vi "Sweep Field and Get Data.vi"(4 "error in":errorcluster, 5 "Spectral Data In":T1={"PDT Amp [v]"=0.0, "RIS Amp [v]"=0.0, "B-Field"=[], "All In-Phase Scan Spectra"=[], "Model Select"=enum."OneCompRISTwoPDT", "Fit Each Scan"=FALSE, "PDT Center [g]"=0.0, "In-Phase Average Spectra"=[], "In-Phase Median Spectra"=[], "Out-Phase Median Spectra"=[], "Out-Phase Average Spectra"=[], "Fit Spectra"=[], "Fit No-Baseline Spectra"=[], "All Out-Phase Scan Spectra"=[], "Baseline Offset Correction"=FALSE, "In-Phase Offset [v]"=0.0, "Out-Phase Offset [v]"=0.0, "Ch2 Input\n(Balance)"=[], "Ch3 Input\n(Phase)"=[], "Ch4 Input\n(AFC)"=[], "Fit Pars"=[], "Fit Pars Errors"=[], "Fit Pars Labels"=[], "Raw Scan DAQ Data"=[], "Bad Scans Indicies"=[], "Good In-Phase Scan Spectra"=[], "Good Out-Phase Scan Spectra"=[], "Bad In-Phase Scan Spectra"=[], "Bad Out-Phase Scan Spectra"=[], "Number of bad scans"=0, "Fit History"=[], "PDT Amp. History/Set [v]"=[], "RIS Amp. History/Set [v]"=[], "RIS Amp. History/Scan [v]"=[], "All Shifted B-Fields"=[], "Good Shifted B-Fields"=[], "Ch5 Input\n(SpO2)"=[], "Ch6 Input\n(BPM)"=[], "Global SNR"=0.0, "Fit Error History"=[], "SNR History"=[]} {"Global SNR" min=0.0; "PDT Center [g]" min=0.0; "RIS Amp [v]" min=0.0; "PDT Amp [v]" min=0.0}, 6 "Hardware Parameters":T3={"Scan Calibration [G/V]"=0.0, "Modulation Calibration [G/V]"=0.0, "Modulation Phase [deg]"=0.0, "Modulation Frequency [Hz]"=0.0, "Attenuation [dB]"=0, "Input Channel Count"=0, "Time constant"=7, "Sensitivity"=17, "Frequency Output Voltage [V]"=0.0, "Phase Output Voltage [V]"=0.0, "Lock-in Offset Compensation"=FALSE, "RF [GHz]"=0.0, "Q Start"=0.0, "Q End"=0.0, "Balance"=0.0, "Phase Error"=0.0, "AFC Error"=0.0, "AFC"=FALSE, "Magnet Rotation"=FALSE, "Balance Scaling Factor"=1.0, "Phase Error Scaling Factor"=1.0, "AFC Error Scaling Factor"=1.0, "Frequency Counter ID"="", "Sweep Waveform"=enum."Sawtooth", "Q-Factor Scale"=0.0, " Q-Data Scale"=0.0, " Q-Data Offset"=0.0, "Magnet Rotation Slope"=0.0, "Magnet Rotation Offset"=0.0, "Phase Sweep Resolution"=0.0, "Hardware Version Number"="", "Spectrometer ID Number"=0, "Spectrometer Name"="", "Lock in Saturation"=0.0, "Balance Threshold"=0.0, "Phase Error Threshold"=0.0, "AFC Error Threshold"=0.0, "Linear Actuator Length"=0.0, "Lock-in OK?"=FALSE, "Ignore Lock-in Comm. Failure"=FALSE, "Gradient Addresses"=[], "Gradient Calibrations [G/A*mm]"=[], "Gradient Power Supplies"=[], "Lock-in Address"="", "Magnet Type"=enum."RRI", "Camera Names"=[], "Sweep Limit [Gauss]"=0.0, "Modulation Limit [Gauss]"=0.0, "Balance Threshold Exceeded?"=FALSE, "Phase Threshold Exceeded?"=FALSE, "AFC Threshold Exceeded?"=FALSE, "Consecutive Re-tune attempts"=0, "Reverse Sweep Slope [sec]"=0.0, "Reverse Sweep Offset [G]"=0.0, "AFC Field Correction [V/MHz]"=0.0, "Active Gradients (X Y Z)"=[], "SpO2 Calibration [SpO2/V]"=1.0, "Heart Rate Calibration [BPM/V]"=1.0, "Thermocouple Channel"=""} {"Sensitivity" items=["10 us", "20 us", "40 us", "80 us", "160 us", "320 us", "640 us", "5 ms", "10 ms", "20 ms", "50 ms", "100 ms", "200 ms", "500 ms", "1 s", "2 s", "5 s", "10 s", "20 s", "50 s", "100 s", "200 s", "500 s", "1 ks", "2 ks", "5 ks", "10 ks", "20 ks", "50 ks", "100 ks"]; "Time constant" items=["10 us", "20 us", "40 us", "80 us", "160 us", "320 us", "640 us", "5 ms", "10 ms", "20 ms", "50 ms", "100 ms", "200 ms", "500 ms", "1 s", "2 s", "5 s", "10 s", "20 s", "50 s", "100 s", "200 s", "500 s", "1 ks", "2 ks", "5 ks", "10 ks", "20 ks", "50 ks", "100 ks"]}, 7 "Acquisition Parameters":T4={"Magnet Angle [deg]"=0.0, "Magnet Angles [deg]"=[], "DeltaVpp [v]"=0.0, "SEM [v]"=0.0, "DeltaVpp Thresh [v]"=0.0, "SEM Thresh [v]"=0.0, "Adaptive Processing"=FALSE, "Acquire Q"=FALSE, "Acquire Photos"=FALSE, "Adaptive Tuning"=FALSE, "Automated Matching"=FALSE, "X-Gradient [G/mm]"=0.0, "Y-Gradient [G/mm]"=0.0, "Z-Gradient [G/mm]"=0.0, "Central Field [G]"=0.0, "Scan Width [G]"=0.0, "Mod. Amp. [G]"=0.0, "Scan Time [s]"=0.0, "Pre-Scan Delay [ms]"=0, "Measurement Timeout [s]"=0.0, "Electromagnet Main Field [G]"=0.0, "Locked Central Field [G]"=0.0, "Scans Excluded"=0, "Scans Completed"=0, "No. Scans/Set"=0, "No. Scans for SNR"=0, "Field Locked Frequency [GHz]"=0.0, "Auto Set-based Field Center"=FALSE, "Prompt for oxy acquisition updates"=FALSE, "Oxy QA Scan?"=FALSE, "Exclude Bad Data"=FALSE, "Optimizing RF Power"=FALSE, "Gradients on/off"=FALSE, "Running Script"=TRUE, "Opto-Coupler Current [A]"=0.0, "Continuous Sweeping"=FALSE, "Sweep Rise Time [sec]"=0, "Reverse Sweep Central Field [G]"=0.0, "Forward Sweep Central Field [G]"=0.0, "Sweep Calibrated"=FALSE, "Modulation Calibrated"=FALSE, "First CheckCal Scan?"=FALSE, "AFC Field Correction"=FALSE, "OxyQAInit Scan Width [G]"=0.0, "OxyQAInit Mod. Amp. [G]"=0.0, "Scans Completed/Session"=0, "Acquire SpO2"=FALSE, "Acquire Temperature"=FALSE, "Over Mod"=FALSE} {"OxyQAInit Mod. Amp. [G]" min=0.0; "OxyQAInit Scan Width [G]" min=0.0; "Mod. Amp. [G]" min=0.0; "Scan Width [G]" min=0.0; "Central Field [G]" min=0.0; "Measurement Timeout [s]" min=0.0; "Scan Time [s]" min=0.0; "Z-Gradient [G/mm]" min=0.0; "SEM [v]" min=0.0; "DeltaVpp [v]" min=0.0}) -> (0 "error out":errorcluster, 2 "Raw DAQ Data Out":dbl[][](array[numeric]), 3 "Spectral Data Out":T1={"PDT Amp [v]"=0.0, "RIS Amp [v]"=0.0, "B-Field"=[], "All In-Phase Scan Spectra"=[], "Model Select"=enum."OneCompRISTwoPDT", "Fit Each Scan"=FALSE, "PDT Center [g]"=0.0, "In-Phase Average Spectra"=[], "In-Phase Median Spectra"=[], "Out-Phase Median Spectra"=[], "Out-Phase Average Spectra"=[], "Fit Spectra"=[], "Fit No-Baseline Spectra"=[], "All Out-Phase Scan Spectra"=[], "Baseline Offset Correction"=FALSE, "In-Phase Offset [v]"=0.0, "Out-Phase Offset [v]"=0.0, "Ch2 Input\n(Balance)"=[], "Ch3 Input\n(Phase)"=[], "Ch4 Input\n(AFC)"=[], "Fit Pars"=[], "Fit Pars Errors"=[], "Fit Pars Labels"=[], "Raw Scan DAQ Data"=[], "Bad Scans Indicies"=[], "Good In-Phase Scan Spectra"=[], "Good Out-Phase Scan Spectra"=[], "Bad In-Phase Scan Spectra"=[], "Bad Out-Phase Scan Spectra"=[], "Number of bad scans"=0, "Fit History"=[], "PDT Amp. History/Set [v]"=[], "RIS Amp. History/Set [v]"=[], "RIS Amp. History/Scan [v]"=[], "All Shifted B-Fields"=[], "Good Shifted B-Fields"=[], "Ch5 Input\n(SpO2)"=[], "Ch6 Input\n(BPM)"=[], "Global SNR"=0.0, "Fit Error History"=[], "SNR History"=[]} {"Global SNR" min=0.0; "PDT Center [g]" min=0.0; "RIS Amp [v]" min=0.0; "PDT Amp [v]" min=0.0})   [LabVIEW 2016]
uses:
  Types/Acquisition Parameters.ctl
  Types/Hardware Parameters.ctl
  Types/Spectral Data.ctl
  Types/Fitting Model Selection.ctl
  Das16.llb/FromEng(single).VI
  Types/Global Variables.vi
  Das16.llb/ToEng(array).vi
panel:
  out "B-Field Out":dbl[](array[numeric])
  # "Bridge I/O"
  # "Magnet Rotation"
  # "Field Calibration"
  # "Lock In Amplifier"
  # "Spectrometer Information"
  # "DAQ Settings"
  # "Gradient Coils and Field"
  # "X"
  # "Y"
  # "Z"
  # "Q-Measurements"
  # "Gradients"
  # "Field"
  # "Scans and Sets"
  # "Timing"
  # "Adaptive Dosimetric \nData Processing"
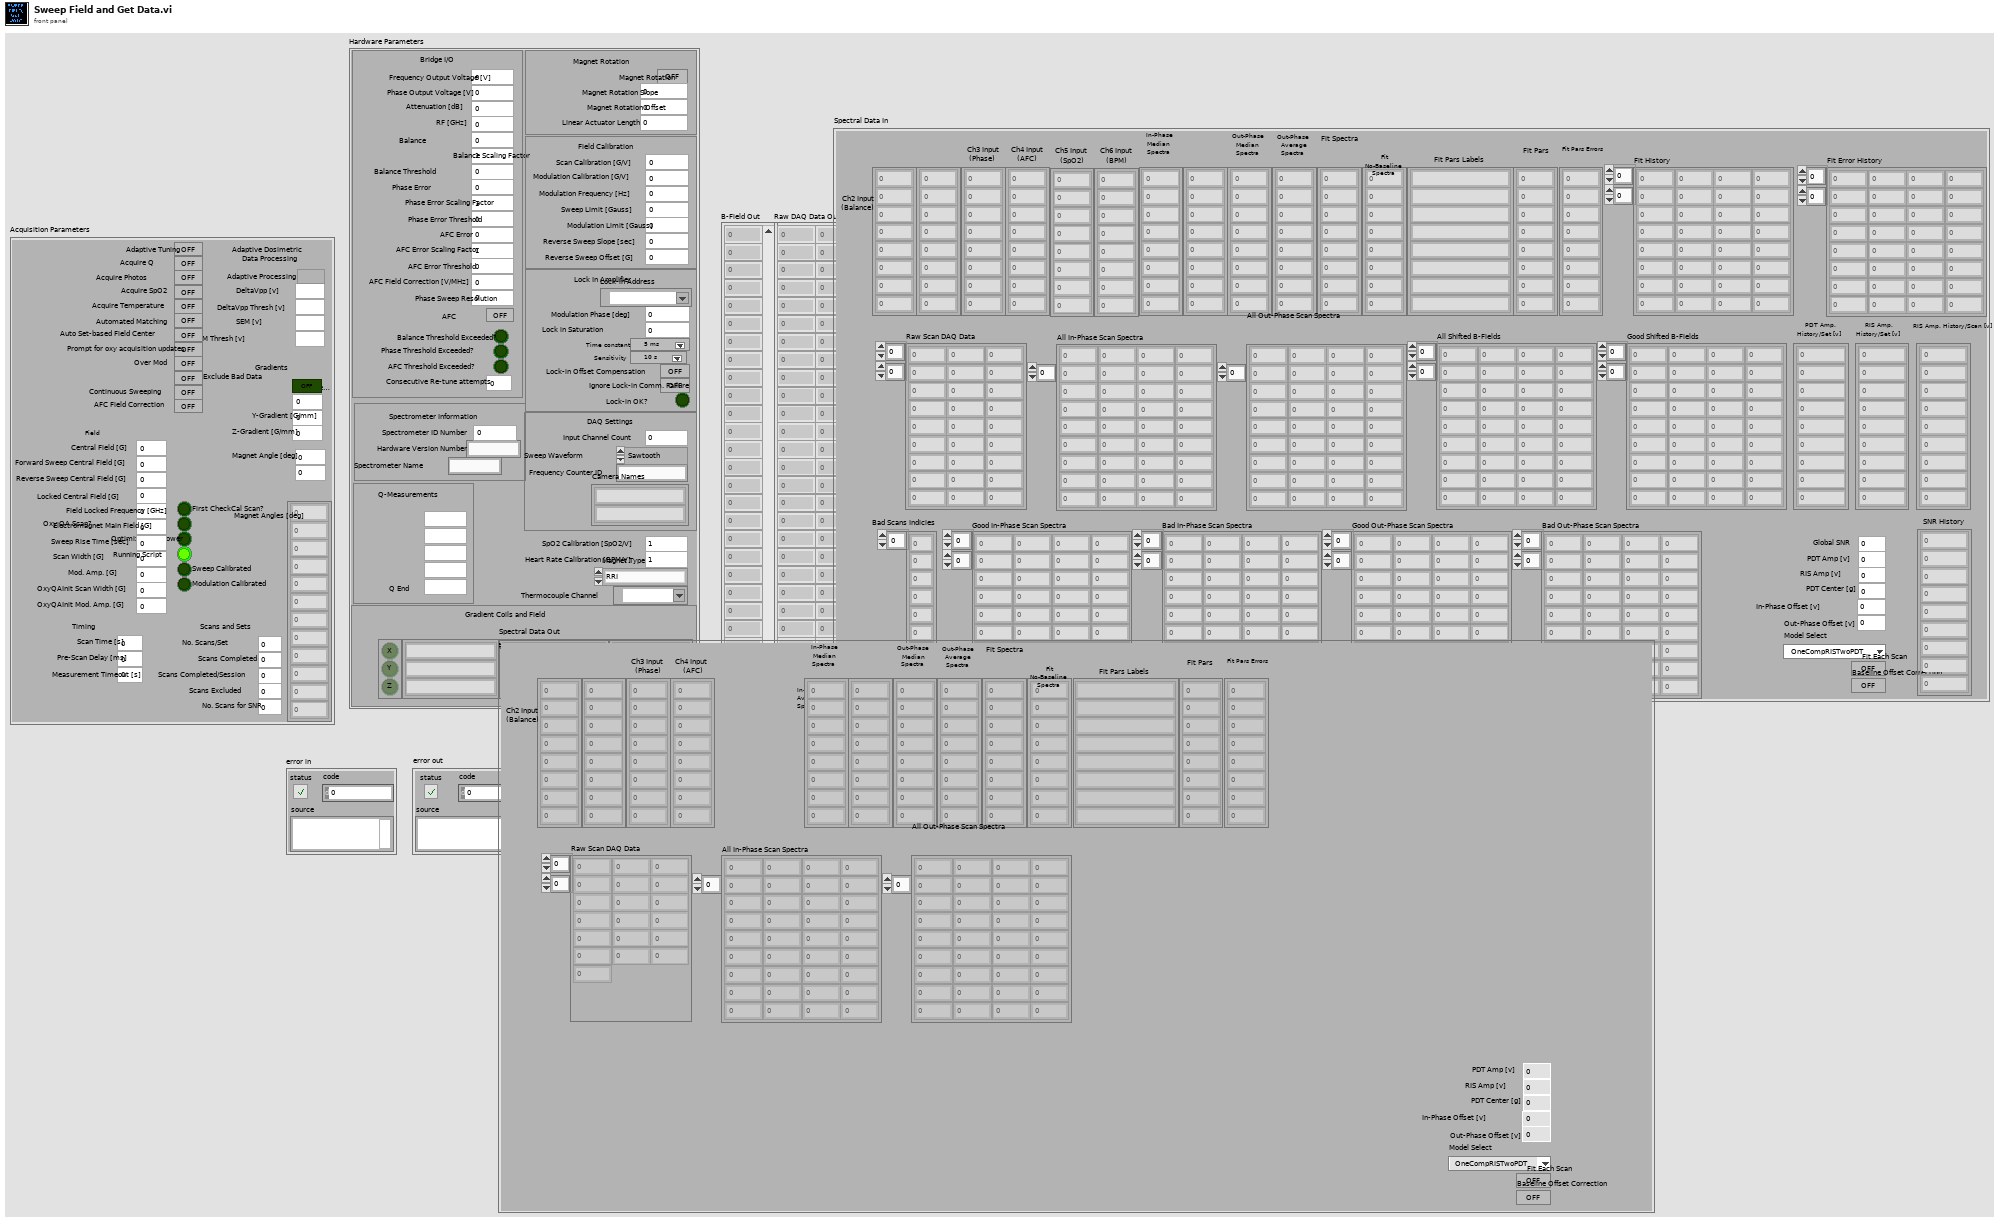
[diagram p1: front panel]
types:
  T1 = typedef "Spectral Data.ctl" = cluster{"PDT Amp [v]":dbl, "RIS Amp [v]":dbl, "B-Field":dbl[], "All In-Phase Scan Spectra":dbl[][], "Model Select":T2, "Fit Each Scan":bool, "PDT Center [g]":dbl, "In-Phase Average Spectra":dbl[], "In-Phase Median Spectra":dbl[], "Out-Phase Median Spectra":dbl[], "Out-Phase Average Spectra":dbl[], "Fit Spectra":dbl[], "Fit No-Baseline Spectra":dbl[], "All Out-Phase Scan Spectra":dbl[][], "Baseline Offset Correction":bool, "In-Phase Offset [v]":dbl, "Out-Phase Offset [v]":dbl, "Ch2 Input\n(Balance)":dbl[], "Ch3 Input\n(Phase)":dbl[], "Ch4 Input\n(AFC)":dbl[], "Fit Pars":dbl[], "Fit Pars Errors":dbl[], "Fit Pars Labels":string[], "Raw Scan DAQ Data":dbl[][], "Bad Scans Indicies":i32[], "Good In-Phase Scan Spectra":dbl[][], "Good Out-Phase Scan Spectra":dbl[][], "Bad In-Phase Scan Spectra":dbl[][], "Bad Out-Phase Scan Spectra":dbl[][], "Number of bad scans":i32, "Fit History":dbl[][], "PDT Amp. History/Set [v]":dbl[], "RIS Amp. History/Set [v]":dbl[], "RIS Amp. History/Scan [v]":dbl[], "All Shifted B-Fields":dbl[][], "Good Shifted B-Fields":dbl[][], "Ch5 Input\n(SpO2)":dbl[], "Ch6 Input\n(BPM)":dbl[], "Global SNR":dbl, "Fit Error History":dbl[][], "SNR History":dbl[]}
  T2 = typedef "Fitting Model Selection.ctl" = enum16{"OneCompRIS", "OneCompRISTwoPDT", "OneCompRISRev", "OneCompRISTwoPDTRev", "LiPc", "TwoLiPc", "ThreeLiPc", "FourLiPc", "PDTCalibration", "CE_Ink", "Printex", "MelaninTwoPDT"}
  T3 = typedef "Hardware Parameters.ctl" = cluster{"Scan Calibration [G/V]":dbl, "Modulation Calibration [G/V]":dbl, "Modulation Phase [deg]":dbl, "Modulation Frequency [Hz]":dbl, "Attenuation [dB]":u16, "Input Channel Count":i32, "Time constant":u16, "Sensitivity":u16, "Frequency Output Voltage [V]":dbl, "Phase Output Voltage [V]":dbl, "Lock-in Offset Compensation":bool, "RF [GHz]":dbl, "Q Start":dbl, "Q End":dbl, "Balance":dbl, "Phase Error":dbl, "AFC Error":dbl, "AFC":bool, "Magnet Rotation":bool, "Balance Scaling Factor":dbl, "Phase Error Scaling Factor":dbl, "AFC Error Scaling Factor":dbl, "Frequency Counter ID":string, "Sweep Waveform":enum16{"Sine Wave", "Square Wave", "Sawtooth", "Triangle Wave"}, "Q-Factor Scale":dbl, " Q-Data Scale":dbl, " Q-Data Offset":dbl, "Magnet Rotation Slope":dbl, "Magnet Rotation Offset":dbl, "Phase Sweep Resolution":dbl, "Hardware Version Number":string, "Spectrometer ID Number":i32, "Spectrometer Name":string, "Lock in Saturation":dbl, "Balance Threshold":dbl, "Phase Error Threshold":dbl, "AFC Error Threshold":dbl, "Linear Actuator Length":dbl, "Lock-in OK?":bool, "Ignore Lock-in Comm. Failure":bool, "Gradient Addresses":string[], "Gradient Calibrations [G/A*mm]":dbl[], "Gradient Power Supplies":string[], "Lock-in Address":refnum<visa-resource-name>, "Magnet Type":enum16{"RRI", "BARDA", "Whole Body Permanent", "RRI Electromagnet"}, "Camera Names":string[], "Sweep Limit [Gauss]":dbl, "Modulation Limit [Gauss]":dbl, "Balance Threshold Exceeded?":bool, "Phase Threshold Exceeded?":bool, "AFC Threshold Exceeded?":bool, "Consecutive Re-tune attempts":i32, "Reverse Sweep Slope [sec]":dbl, "Reverse Sweep Offset [G]":dbl, "AFC Field Correction [V/MHz]":dbl, "Active Gradients (X Y Z)":bool[], "SpO2 Calibration [SpO2/V]":dbl, "Heart Rate Calibration [BPM/V]":dbl, "Thermocouple Channel":tag}
  T4 = typedef "Acquisition Parameters.ctl" = cluster{"Magnet Angle [deg]":dbl, "Magnet Angles [deg]":dbl[], "DeltaVpp [v]":dbl, "SEM [v]":dbl, "DeltaVpp Thresh [v]":dbl, "SEM Thresh [v]":dbl, "Adaptive Processing":bool, "Acquire Q":bool, "Acquire Photos":bool, "Adaptive Tuning":bool, "Automated Matching":bool, "X-Gradient [G/mm]":dbl, "Y-Gradient [G/mm]":dbl, "Z-Gradient [G/mm]":dbl, "Central Field [G]":dbl, "Scan Width [G]":dbl, "Mod. Amp. [G]":dbl, "Scan Time [s]":dbl, "Pre-Scan Delay [ms]":u32, "Measurement Timeout [s]":dbl, "Electromagnet Main Field [G]":dbl, "Locked Central Field [G]":dbl, "Scans Excluded":u32, "Scans Completed":u32, "No. Scans/Set":u32, "No. Scans for SNR":u32, "Field Locked Frequency [GHz]":dbl, "Auto Set-based Field Center":bool, "Prompt for oxy acquisition updates":bool, "Oxy QA Scan?":bool, "Exclude Bad Data":bool, "Optimizing RF Power":bool, "Gradients on/off":bool, "Running Script":bool, "Opto-Coupler Current [A]":dbl, "Continuous Sweeping":bool, "Sweep Rise Time [sec]":u32, "Reverse Sweep Central Field [G]":dbl, "Forward Sweep Central Field [G]":dbl, "Sweep Calibrated":bool, "Modulation Calibrated":bool, "First CheckCal Scan?":bool, "AFC Field Correction":bool, "OxyQAInit Scan Width [G]":dbl, "OxyQAInit Mod. Amp. [G]":dbl, "Scans Completed/Session":u32, "Acquire SpO2":bool, "Acquire Temperature":bool, "Over Mod":bool}
  T5 = enum16{"Sine Wave", "Square Wave", "Sawtooth", "Triangle Wave"}
  T6 = cluster{"IntnlBoardNum":i32, "Data":i16[], "Size":i32, "IntnlStatus":i32, "IntnlErrCode":i32, "Alias16":u32, "Reserved":i32}
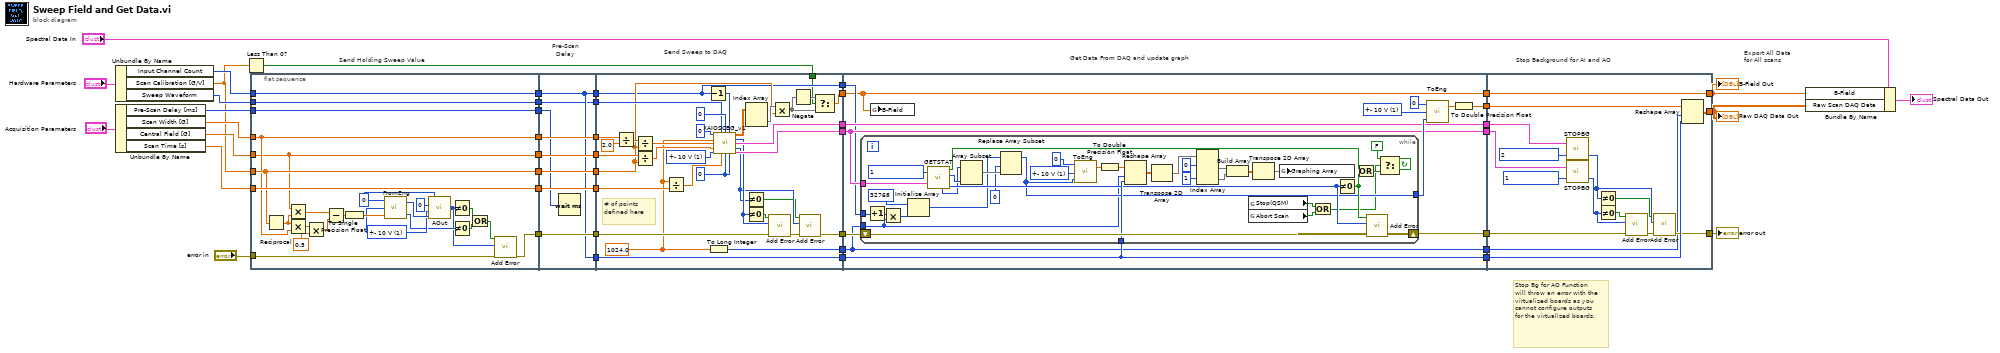
[diagram p0: block diagram]
diagram:
  # "Stop Background for AI and AO"
  # "Get Data From DAQ and update graph"
  # "Send Holding Sweep Value"
  # "Pre-Scan\n  Delay"
  # "Send Sweep to DAQ"
  # "Stop Bg for AO Function will throw an error with the virtualized boards as you cannot configure outputs for the virtualized boards."
  # "Export All Data \nfor All scans"
  n1 = Unbundle By Name("Hardware Parameters") -> ("Input Channel Count"=w16:i32, "Scan Calibration [G/V]"=w2:dbl, "Sweep Waveform"=w12:T5)
  n2 = Unbundle By Name("Acquisition Parameters") -> ("Pre-Scan Delay [ms]"=w17:u32, "Scan Width [G]"=w15:dbl, "Central Field [G]"=w14:dbl, "Scan Time [s]"=w13:dbl)
  n3 = Less Than 0?(x=w2) -> (x < 0?=w1:bool)
  n4 = flat-sequence {
    tunnel: w13 -> [w70]
    tunnel: w14 -> [w62]
    tunnel: w15 -> [w63]
    tunnel: w2 -> [w64]
    tunnel: "error in" -> [w54]
    tunnel: w16 -> [w71]
    tunnel: [w71] -> w46
    tunnel: [w52] -> w45
    tunnel: [w64] -> w44
    tunnel: [w63] -> w43
    tunnel: [w62] -> w42
    tunnel: [w70] -> w41
    tunnel: w17 -> [w53]
    tunnel: [w53] -> w40
    tunnel: w12 -> [w47]
    tunnel: [w47] -> w10
    tunnel: w46 -> [w73]
    tunnel: [w73] -> w39
    tunnel: w45 -> [w79]
    tunnel: [w79] -> w38
    tunnel: w44 -> [w78]
    tunnel: [w78] -> w37
    tunnel: w43 -> [w77]
    tunnel: [w77] -> w36
    tunnel: w42 -> [w76]
    tunnel: [w76] -> w35
    tunnel: w41 -> [w75]
    tunnel: [w75] -> w34
    tunnel: w40 -> [w74]
    tunnel: [w73] -> w33
    tunnel: [w72] -> w11
    tunnel: w10 -> [w72]
    tunnel: [w103] -> w32
    tunnel: [w102] -> w31
    tunnel: w39 -> [w86]
    tunnel: w38 -> [w97]
    tunnel: w37 -> [w87]
    tunnel: w36 -> [w101]
    tunnel: w35 -> [w100]
    tunnel: w34 -> [w99]
    tunnel: w33 -> [w98]
    tunnel: [w98] -> w30
    tunnel: [w93] -> w29
    tunnel: [w83] -> w28
    tunnel: w11 -> [w89]
    tunnel: [w86] -> w9
    tunnel: [w84] -> w8
    tunnel: w1 -> [w80]
    tunnel: w32 -> [w123]
    tunnel: w31 -> [w122]
    tunnel: [w123] -> w27
    tunnel: [w122] -> w26
    tunnel: [w117] -> w25
    tunnel: [w119] -> w24
    tunnel: w30 -> [w118]
    tunnel: [w118] -> w23
    tunnel: w29 -> [w121]
    tunnel: [w115] -> w22
    tunnel: w28 -> [w115]
    tunnel: w9 -> [w116]
    tunnel: w8 -> [w114]
    tunnel: [w114] -> w7
    tunnel: w27 -> [w179]
    tunnel: w26 -> [w178]
    tunnel: w25 -> [w173]
    tunnel: w24 -> [w175]
    tunnel: w23 -> [w172]
    tunnel: w22 -> [w165]
    tunnel: w7 -> [w164]
    tunnel: [w165] -> w5
    tunnel: [w174] -> w3
    tunnel: [w169] -> w20
    frame #0 {
      w56 = 1 items=["Not Programmable"=0, "+- 20 V"=27, "+- 10 V"=1, "+- 5 V"=2, "+- 4 V"=28, "+- 2.5 V"=3, "+- 2 V"=29, "+- 1.67 V"=4, "+- 1.25 V"=5, "+- 1 V"=6, "+- .625 V"=7, "+- .5 V"=8, "+- .25 V"=30, "+- .2 V"=31, "+- .1 V"=9, "+- .05 V"=10, "+- .01 V"=11, "+- .005 V"=12, "0 - 10 V"=13, "0 - 5 V"=14, "0 - 4 V"=36, "0 - 2.5 V"=15, "0 - 2 V"=16, "0 - 1.67 V"=17, "0 - 1.25 V"=18, "0 - 1 V"=19, "0 - .5 V"=32, "0 - .25 V"=33, "0 - .2 V"=34, "0 - .1 V"=20, "0 - .02 V"=35, "0 - .01 V"=21, "4 - 20 mA"=22, "2 - 10 mA"=23, "1 - 5 mA"=24, ".5 - 2.5 mA"=25, "0 - 20 mA"=26] ("Range")
      w58 = u32 0 ("BoardNum (0)")
      n5 = Reciprocal(x=w64) -> (1/x=w69:dbl)
      n6 = Multiply(x=w62, y=w69) -> (x*y=w65:dbl)
      n7 = Multiply(x=w69, y=w63) -> (x*y=w68:dbl)
      n8 = Multiply(x=w68, y=0.5) -> (x*y=w66:dbl)
      n9 = Subtract(x=w65, y=w66) -> (x-y=w60:dbl)
      n10 = To Single Precision Float(number=w60) -> (single precision float=w61:sgl)
      n11 = call-poly "FromEng.VI"("Eng Units"=w61, "Range"=w56, "BoardNum (0)"=w58) -> ("ErrCode"=w55:i32, "DA Data"=w57:u16)
      n12 = call "AOut.VI"("DataValue"=w57, "Range"=w56, "Channel"=0, "BoardNum"=w58) -> ("ErrCode"=w48:i32)
      n13 = Not Equal To 0?(x=w48) -> (x != 0?=w49:bool)
      n14 = Not Equal To 0?(x=w55) -> (x != 0?=w51:bool)
      n15 = Or(x=w49, y=w51) -> (x .or. y?=w50:bool)
      n16 = call "Add Error.vi"("error in (no error)"=w54, "error code (0)"=w48, "error?"=w50) -> ("error out"=w52:errorcluster)  [unwired: 8 in]
    }
    frame #1 {
      n17 = Wait (ms)(milliseconds to wait=w74) -> ()  [unwired: 1 out]
    }
    frame #2 {
      w85 = 1024.0 ("y")
      w104 = 0 ("LowAOChan")
      w112 = 1 items=["Not Programmable"=0, "+- 20 V"=27, "+- 10 V"=1, "+- 5 V"=2, "+- 4 V"=28, "+- 2.5 V"=3, "+- 2 V"=29, "+- 1.67 V"=4, "+- 1.25 V"=5, "+- 1 V"=6, "+- .625 V"=7, "+- .5 V"=8, "+- .25 V"=30, "+- .2 V"=31, "+- .1 V"=9, "+- .05 V"=10, "+- .01 V"=11, "+- .005 V"=12, "0 - 10 V"=13, "0 - 5 V"=14, "0 - 4 V"=36, "0 - 2.5 V"=15, "0 - 2 V"=16, "0 - 1.67 V"=17, "0 - 1.25 V"=18, "0 - 1 V"=19, "0 - .5 V"=32, "0 - .25 V"=33, "0 - .2 V"=34, "0 - .1 V"=20, "0 - .02 V"=35, "0 - .01 V"=21, "4 - 20 mA"=22, "2 - 10 mA"=23, "1 - 5 mA"=24, ".5 - 2.5 mA"=25, "0 - 20 mA"=26] ("Range")
      # "# of points defined here"
      n18 = Divide(x=w101, y=2.0) -> (x/y=w108:dbl)
      n19 = Divide(x=w108, y=w87) -> (x/y=w107:dbl)
      n20 = Divide(x=w100, y=w87) -> (x/y=w106:dbl)
      n21 = Divide(x=w85, y=w99) -> (x/y=w105:dbl)
      n22 = Decrement(x=w86) -> (x-1=w111:i32)
      n23 = To Long Integer(number=w85) -> (32bit integer=w84:i32)
      n24 = call "XAIOSCBG_v1.VI"("BoardNum"=u32 0, "signal type"=w89, "LowChan"=0, "HighChan"=w111, "number of points"=w85, "amplitude (1.0)"=w107, "offset (0.0)"=w106, "Range"=w112, "Rate"=w105, "HighAOChan"=w104, "LowAOChan"=w104) -> ("Output Array"=w90:dbl[][], "AIn-ErrCode"=w96:i32, "OutContext"=w103:T6, "AOut-ErrCode"=w95:i32, "InContext"=w102:T6)
      n25 = Not Equal To 0?(x=w95) -> (x != 0?=w92:bool)
      n26 = Not Equal To 0?(x=w96) -> (x != 0?=w91:bool)
      n27 = Index Array(array=w90) -> (element=w88:dbl[])  [unwired: 2 in]
      n28 = call "Add Error.vi"("error in (no error)"=w97, "error code (0)"=w96, "error?"=w91) -> ("error out"=w94:errorcluster)  [unwired: 8 in]
      n29 = Multiply(x=w88, y=w87) -> (x*y=w82:dbl[])
      n30 = Negate(x=w82) -> (-x=w81:dbl[])
      n31 = call "Add Error.vi"("error in (no error)"=w94, "error code (0)"=w95, "error?"=w92) -> ("error out"=w93:errorcluster)  [unwired: 8 in]
      n32 = Select(t=w81, s=w80, f=w82) -> (s? t:f=w83:dbl[])
    }
    frame #3 {
      w125 = 1 items=["Not Programmable"=0, "+- 20 V"=27, "+- 10 V"=1, "+- 5 V"=2, "+- 4 V"=28, "+- 2.5 V"=3, "+- 2 V"=29, "+- 1.67 V"=4, "+- 1.25 V"=5, "+- 1 V"=6, "+- .625 V"=7, "+- .5 V"=8, "+- .25 V"=30, "+- .2 V"=31, "+- .1 V"=9, "+- .05 V"=10, "+- .01 V"=11, "+- .005 V"=12, "0 - 10 V"=13, "0 - 5 V"=14, "0 - 4 V"=36, "0 - 2.5 V"=15, "0 - 2 V"=16, "0 - 1.67 V"=17, "0 - 1.25 V"=18, "0 - 1 V"=19, "0 - .5 V"=32, "0 - .25 V"=33, "0 - .2 V"=34, "0 - .1 V"=20, "0 - .02 V"=35, "0 - .01 V"=21, "4 - 20 mA"=22, "2 - 10 mA"=23, "1 - 5 mA"=24, ".5 - 2.5 mA"=25, "0 - 20 mA"=26] ("Range")
      n33 = while {
        tunnel: w122 -> [w163]
        tunnel: [w144] -> w126
        shift-right: [w160] -> w117
        shift-left: w121 -> [w161]
        tunnel: w118 -> [w154]
        tunnel: w116 -> [w142]
        tunnel: w114 -> [w138]
        stop <- w153 continue-if-true
        w145 = 1 items=["Not Programmable"=0, "+- 20 V"=27, "+- 10 V"=1, "+- 5 V"=2, "+- 4 V"=28, "+- 2.5 V"=3, "+- 2 V"=29, "+- 1.67 V"=4, "+- 1.25 V"=5, "+- 1 V"=6, "+- .625 V"=7, "+- .5 V"=8, "+- .25 V"=30, "+- .2 V"=31, "+- .1 V"=9, "+- .05 V"=10, "+- .01 V"=11, "+- .005 V"=12, "0 - 10 V"=13, "0 - 5 V"=14, "0 - 4 V"=36, "0 - 2.5 V"=15, "0 - 2 V"=16, "0 - 1.67 V"=17, "0 - 1.25 V"=18, "0 - 1 V"=19, "0 - .5 V"=32, "0 - .25 V"=33, "0 - .2 V"=34, "0 - .1 V"=20, "0 - .02 V"=35, "0 - .01 V"=21, "4 - 20 mA"=22, "2 - 10 mA"=23, "1 - 5 mA"=24, ".5 - 2.5 mA"=25, "0 - 20 mA"=26] ("Range")
        n34 = Increment(x=w142) -> (x+1=w141:i32)
        n35 = Multiply(x=w141, y=w138) -> (x*y=w140:i32)
        n36 = Initialize Array(u16 32768 ("Y-default"), w140) -> (w143:u16[])
        n37 = call "GETSTAT.VI"("Function Type"=1, "Context"=w163) -> ("Data"=w148:u16[], "Running"=w159:bool, "CurCount"=w149:i32, "ErrCode"=w150:i32)  [unwired: 2 out]
        n38 = Array Subset(array=w148, length=w149) -> (w147:u16[])  [unwired: 1 in]
        n39 = Replace Array Subset(array=w143, new element=w147, index=0) -> (w144:u16[])
        n40 = call-poly "ToEng.VI"("AD Data"=w144, "Range"=w145, "BoardNum"=u32 0) -> ("Eng Units"=w156:sgl[])  [unwired: 1 out]
        n41 = To Double Precision Float(number=w156) -> (double precision float=w155:dbl[])
        n42 = Reshape Array(w155, w138, w154) -> (w133:dbl[][])
        n43 = Transpose 2D Array(2D array=w133) -> (transposed array=w132:dbl[][])
        n44 = Index Array(array=w132, index (row) #1=0 ("index (row)"), index (row) #2=1 ("index (row)")) -> (element #1=w135:dbl[], element #2=w134:dbl[])  [unwired: 2 in]
        n45 = Build Array(w135, w134) -> (w131:dbl[][])
        n46 = global read "Global Variables.vi" "Stop(QSM)"() -> (w128:bool)
        n47 = global read "Global Variables.vi" "Abort Scan"() -> (w129:bool)
        n48 = Transpose 2D Array(2D array=w131) -> (transposed array=w130:dbl[][])
        n49 = global write "Global Variables.vi" "Graphing Array"(w130) -> ()
        n50 = Or(x=w128, y=w129) -> (x .or. y?=w127:bool)
        n51 = Not Equal To 0?(x=w150) -> (x != 0?=w158:bool)
        n52 = Or(x=w159, y=w158) -> (x .or. y?=w152:bool)
        n53 = call "Add Error.vi"("error in (no error)"=w161, "error code (0)"=w150, "error?"=w158) -> ("error out"=w160:errorcluster)  [unwired: 8 in]
        n54 = Select(t=FALSE, s=w127, f=w152) -> (s? t:f=w153:bool)
      }
      n55 = global write "Global Variables.vi" "B-Field"(w115) -> ()
      n56 = call-poly "ToEng.VI"("AD Data"=w126, "Range"=w125, "BoardNum"=u32 0) -> ("Eng Units"=w120:sgl[])  [unwired: 1 out]
      n57 = To Double Precision Float(number=w120) -> (double precision float=w119:dbl[])
    }
    frame #4 {
      n58 = call "STOPBG.VI"("Function Type"=2, "Context"=w179) -> ("ErrorCode"=w168:i32)  [unwired: 1 out]
      n59 = call "STOPBG.VI"("Function Type"=1, "Context"=w178) -> ("ErrorCode"=w171:i32)  [unwired: 1 out]
      n60 = Not Equal To 0?(x=w168) -> (x != 0?=w166:bool)
      n61 = Not Equal To 0?(x=w171) -> (x != 0?=w167:bool)
      n62 = call "Add Error.vi"("error in (no error)"=w173, "error code (0)"=w171, "error?"=w167) -> ("error out"=w170:errorcluster)  [unwired: 8 in]
      n63 = call "Add Error.vi"("error in (no error)"=w170, "error code (0)"=w168, "error?"=w166) -> ("error out"=w169:errorcluster)  [unwired: 8 in]
      n64 = Reshape Array(w175, w164, w172) -> (w174:dbl[][])
    }
  }
  n65 = Bundle By Name(cluster="Spectral Data In", "B-Field"=w5, "Raw Scan DAQ Data"=w3) -> (→"Spectral Data Out":T1)
  "B-Field Out" <- w5
  "Raw DAQ Data Out" <- w3
  "error out" <- w20
